vi "svfa_Spectrum Peak Tone Search and Estimation (complex).vi"(8 "error in (no error)":errorcluster, 9 "criterion":T1={"Single/Multiple"=enum."Multiple Peaks", "Threshold"=0.0, "advanced search"={"approximate frequencies"=[], "advanced span [Hz]"=5.0}} {"advanced search"."advanced span [Hz]" format="%0.2p"; "Threshold" format="%.2f"}, 11 "complex spectrum":T9={"complex spectrum response"={"f0"=0.0, "df"=1.0, "complex spectrum"=[]}, "spectrum info"={"channel name"="", "description"="", "x-axis units"=0, "spectral info"={"spectrum type"=enum."Power [Magnitude^2]", "linear/dB"=enum."linear", "window"=0, "window size"=0, "FFT size"=0}, "engineering units"=0, "custom label"="", "dB reference [EU]"=0.0, "peak units"=enum."rms", "weighting filter"=0, "spectral density?"=FALSE, "unit label"="", "spectrum skewed?"=FALSE, "complimentary spectrum units"=enum."none"}} {"spectrum info"."x-axis units" items=["Time (s)"=0, "Frequency-CB (Hz)"=1, "Frequency-CPB (Hz)"=1248, "Frequency-Arbitrary (Hz)"=2357, "Quefrency (s)"=2, "Revolutions (rev)"=3, "Order"=4, "Speed (RPM)"=11, "Speed (rad/s)"=21, "Index"=65535]; "spectrum info"."weighting filter" items=["Linear", "A-weighting", "B-weighting", "C-weighting", "ITU-R 468-4", "Dolby", "CCITT", "C-message", "Wb", "Wc", "Wd", "We", "Wf", "Wh", "Wj", "Wk", "Wm", "AES17 20 kHz lowpass", "AES17 40 kHz lowpass", "AES17 20 kHz highpass", "AES17 40 kHz highpass"]; "spectrum info"."dB reference [EU]" format="%.2f"; "spectrum info"."engineering units" items=["custom..."=0, "V"=1, "A"=21, "C"=30, "pC"=31, "s"=32, "-"=29, "Pa"=2, "N"=20, "g"=3, "m/s^2"=4, "m/s"=5, "m"=6, "mm/s"=12, "mm"=13, "micron/s"=14, "micron"=15, "in/s^2"=7, "in/s"=8, "in"=9, "mil/s"=10, "mil"=11, "rad/s^2"=16, "rad/s"=17, "rad"=18, "deg/s^2"=26, "deg/s"=27, "deg"=28, "RPM"=22, "cycle/s^2"=23, "Hz"=24, "cycle"=25, "strain"=19]; "spectrum info"."spectral info"."window" items=["None "=0, "Hanning"=1, "Hamming"=2, "Blackman-Harris"=3, "Exact Blackman"=4, "Blackman"=5, "Flat Top"=6, "4 Term B-Harris "=7, "7 Term B-Harris"=8, "Low Sidelobe"=9, "Force - Exponential"=10, "Gaussian"=62]; "complex spectrum response"."complex spectrum" format="%.2f"; "complex spectrum response"."df" format="%.9f"; "complex spectrum response"."f0" format="%.2f"}) -> (0 "error out":errorcluster, 2 "Number of peaks":i32, 3 "peaks":T2(array[cluster]) {"phase [degree]" format="%.2f"; "magnitude" format="%.4f"; "frequency [Hz]" format="%.2f"})   [LabVIEW 2017]
uses:
  <vilib>/addons/_NISVFA/_Shared subVIs/Controls/svc_Spectrum Info.ctl
  <vilib>/addons/_NISVFA/_Shared subVIs/Controls/svc_X-Axis Units.ctl
  <vilib>/addons/_NISVFA/_Shared subVIs/Controls/svc_Spectrum Type.ctl
  <vilib>/addons/_NISVFA/_Shared subVIs/Controls/svc_Engineering Units Text Ring.ctl
  <vilib>/addons/_NISVFA/_Shared subVIs/Controls/svc_Weighting Filter Text Ring.ctl
  <vilib>/addons/_NISVFA/_Shared subVIs/Controls/svc_Complimentary Spectrum Units.ctl
  <vilib>/Analysis/_algsub.llb/Vector Norm.vi
  <vilib>/Analysis/_algsub.llb/Complex Vector Norm.vi
  <vilib>/addons/_NISVFA/_Spectrum Processing/subVIs/svfa_Tone Estimation (complex).vi
  <vilib>/addons/_NISVFA/_Spectrum Processing/SVFA Get Spectrum Subset.vi
  <vilib>/addons/_NISVFA/_Spectrum Processing/SVFA Get Spectrum Subset (Complex) (1 Ch).vi
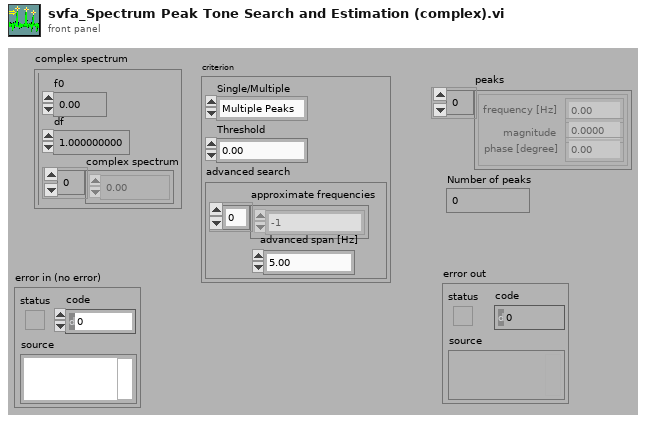
[diagram p1: front panel]
types:
  T1 = cluster{"Single/Multiple":enum16{"Multiple Peaks", "Single Max Peak"}, "Threshold":dbl, "advanced search":cluster{"approximate frequencies":dbl[], "advanced span [Hz]":dbl}}
  T2 = cluster{"frequency [Hz]":dbl, "magnitude":dbl, "phase [degree]":dbl}[]
  T3 = typedef "svc_Spectrum Info.ctl" = cluster{"channel name":string, "description":string, "x-axis units":T4, "spectral info":cluster{"spectrum type":T5, "linear/dB":enum16{"linear", "dB"}, "window":u16, "window size":i32, "FFT size":i32}, "engineering units":T6, "custom label":string, "dB reference [EU]":dbl, "peak units":enum16{"rms", "peak", "peak-peak"}, "weighting filter":T7, "spectral density?":bool, "unit label":string, "spectrum skewed?":bool, "complimentary spectrum units":T8}
  T4 = typedef "svc_X-Axis Units.ctl" = u16
  T5 = typedef "svc_Spectrum Type.ctl" = enum16{"FFT Spectrum [complex]", "Amplitude [Magnitude]", "Power [Magnitude^2]", "Cross Spectrum [complex]", "Frequency Response [Complex]"}
  T6 = typedef "svc_Engineering Units Text Ring.ctl" = u16
  T7 = typedef "svc_Weighting Filter Text Ring.ctl" = u16
  T8 = typedef "svc_Complimentary Spectrum Units.ctl" = enum16{"none", "radians", "degrees", "cycles", "imaginary"}
  T9 = cluster{"complex spectrum response":cluster{"f0":dbl, "df":dbl, "complex spectrum":cdb[]}, "spectrum info":T3}
  T10 = cluster{"frequency [Hz]":dbl, "amplitude":dbl, "phase [degree]":dbl}[]
  T11 = cluster{"frequency [Hz]":dbl, "amplitude":dbl, "phase [degree]":dbl}
  T12 = cluster{"frequency":dbl, "amplitude":dbl, "phase [degree]":dbl}
  T13 = cluster{"frequency [Hz]":dbl, "amplitude [EU pk]":dbl, "phase [deg]":dbl}
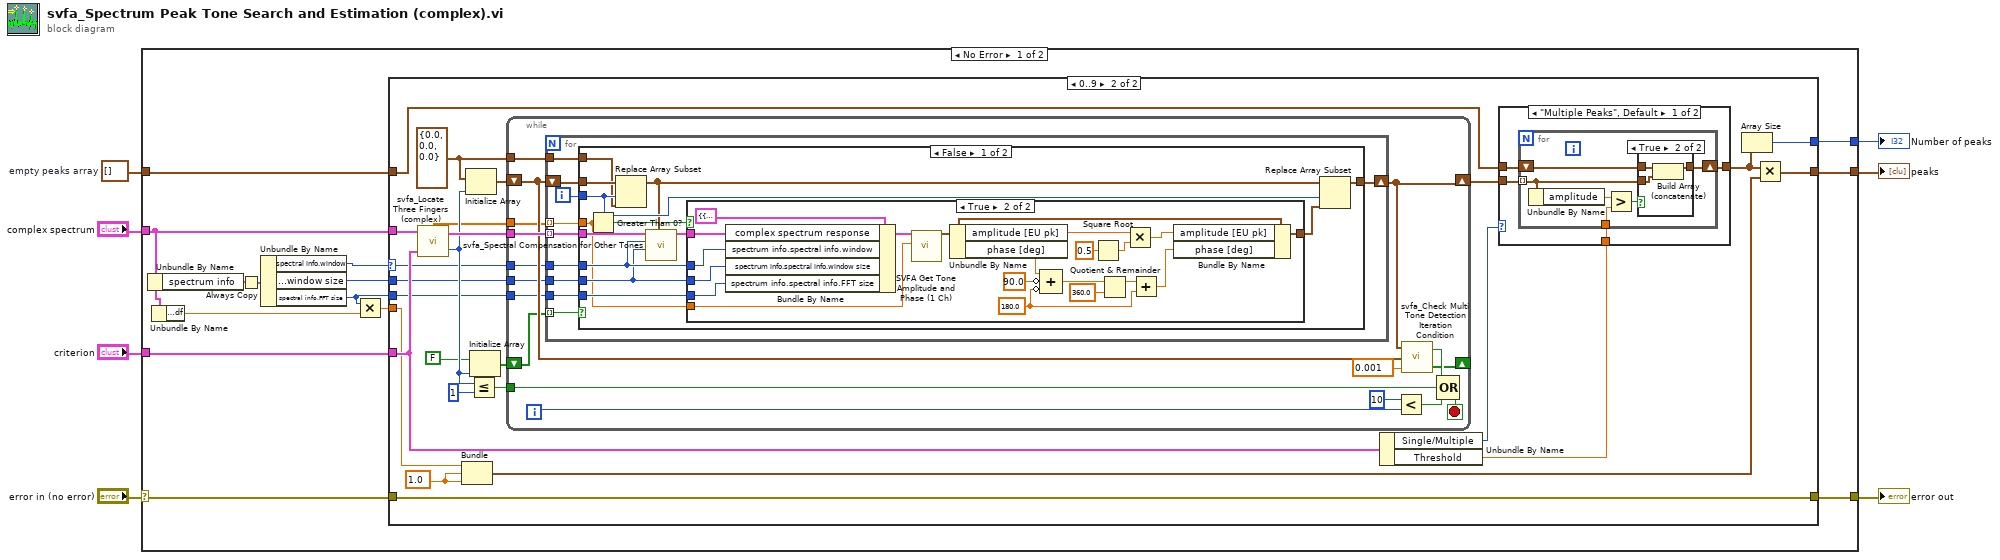
[diagram p0: block diagram]
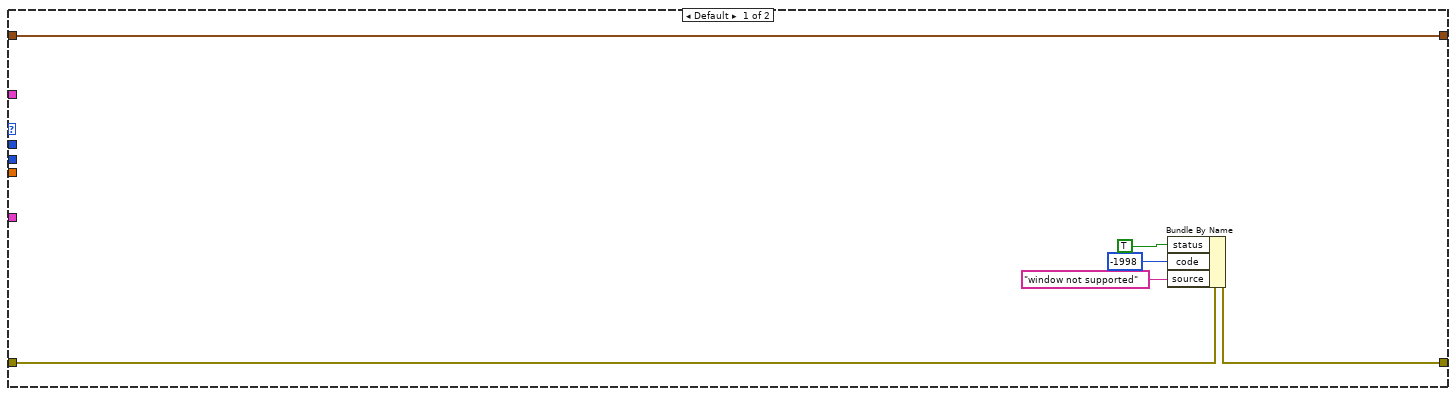
[diagram p2: hidden frame]
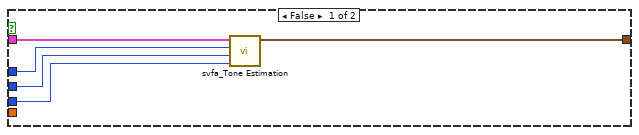
[diagram p3: hidden frame]
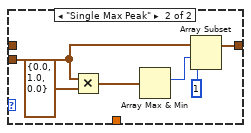
[diagram p6: hidden frame]
diagram:
  w1 = T10 []  # empty peaks array
  n1 = case shown="No Error" "error in (no error)" {
    selector: "error in (no error)" -> [w17 w140]
    tunnel: [w16 w140] -> w6
    tunnel: "criterion" -> [w8 _]
    tunnel: "complex spectrum" -> [w12 _]
    tunnel: [w20 w139] -> w3
    tunnel: [w19 _] -> w2
    tunnel: w1 -> [w9 w139]
    frame No Error {
      n2 = Unbundle By Name(w12) -> ("spectrum info"=w13:T3)
      n3 = Unbundle By Name(w12) -> ("complex spectrum response.df"=w11:dbl)
      n4 = Always Copy(1:w13) -> (0:w10:T3)
      n5 = Unbundle By Name(w10) -> ("spectral info.window"=w18:u16, "spectral info.window size"=w21:i32, "spectral info.FFT size"=w15:i32)
      n6 = Multiply(x=w15, y=w11) -> (x*y=w14:dbl)
      n7 = case shown="0..9" w18 {
        selector: w18 -> [_ w32]
        tunnel: w12 -> [_ w39]
        tunnel: w8 -> [_ w38]
        tunnel: w21 -> [_ w36]
        tunnel: w15 -> [_ w35]
        tunnel: [w22 w34] -> w20
        tunnel: [_ w33] -> w19
        tunnel: w17 -> [w27 w31]
        tunnel: [w23 w31] -> w16
        tunnel: w14 -> [_ w30]
        tunnel: w9 -> [w22 w29]
        frame Default {
          n8 = Bundle By Name(cluster=w27, "status"=TRUE, "code"=-1998, "source"="window not supported") -> (w23:errorcluster)
        }
        frame 0..9 {
          w37 = T11 {"frequency [Hz]"=0.0, "amplitude"=0.0, "phase [degree]"=0.0} ("single tone info.")
          w47 = 1.0 ("x*y")
          n9 = call <vilib>:"svfa_Locate Three Fingers (complex).vi"("criterion"=w38, "complex spectrum"=w39) -> ("number of tones"=w42:i32, "three fingers (frequency normorlized)"=w52:cluster{"f0":dbl, "df":dbl, "spectrum":cdb[]}[], "exact normalized frequencies?"=w28:dbl[])  [unwired: 1 in]
          n10 = Bundle(w30, "x*y"=w47, "x*y"=w47) -> (w48:cluster{dbl, "x*y":dbl, "x*y":dbl})  [unwired: 1 in]
          n11 = Initialize Array(w37, w42) -> (w51:T10)
          n12 = Less Or Equal?(x=w42, y=1) -> (x <= y?=w49:bool)
          n13 = Initialize Array(FALSE ("all stable?"), w42) -> (w43:bool[])
          n14 = while {
            shift-left: w43 -> [w59]
            shift-right: [w58] -> _
            tunnel: w49 -> [w65]
            shift-left: w51 -> [w67]
            shift-right: [w68] -> w46
            tunnel: w52 -> [w69]
            tunnel: w37 -> [w57]
            tunnel: w32 -> [w56]
            tunnel: w36 -> [w55]
            tunnel: w35 -> [w54]
            tunnel: w28 -> [w53]
            i -> [w63]
            stop <- w61 stop-if-true
            n15 = for {
              tunnel: w69 -> [w78] mode=indexing
              shift-right: [w79] -> w68
              shift-left: w67 -> [w77]
              tunnel: w59 -> [w75] mode=indexing
              tunnel: w57 -> [w74]
              tunnel: w56 -> [w73]
              tunnel: w55 -> [w72]
              tunnel: w54 -> [w71]
              tunnel: w53 -> [w70] mode=indexing
              i -> [w76]
              n16 = case shown="False" w75 {
                tunnel: [w92 w118] -> w79
                tunnel: w78 -> [w91 _]
                tunnel: w77 -> [w90 w118]
                tunnel: w76 -> [w89 _]
                tunnel: w74 -> [w86 _]
                tunnel: w73 -> [w84 _]
                tunnel: w72 -> [w83 _]
                tunnel: w71 -> [w82 _]
                tunnel: w70 -> [w80 _]
                frame False {
                  n17 = Greater Than 0?(x=w80) -> (x > 0?=w81:bool)
                  n18 = Replace Array Subset(array=w90, new element=w86, index=w89) -> (w85:T10)
                  n19 = call <vilib>:"svfa_Spectral Compensation for Other Tones.vi"("other tones' information"=w85, "window size"=w83, "window"=w84, "FFT spectrum"=w91) -> ("compensated FFT spectrum"=w88:cluster{"f0":dbl, "df":dbl, "spectrum":cdb[]})  [unwired: 7 in]
                  n20 = case shown="True" w81 {
                    tunnel: w88 -> [w97 w116]
                    tunnel: [w96 w109] -> w87
                    tunnel: w84 -> [w95 w115]
                    tunnel: w83 -> [w94 w114]
                    tunnel: w82 -> [w93 w113]
                    tunnel: w80 -> [_ w111]
                    frame False {
                      n21 = call-poly <vilib>:"svfa_Tone Estimation.vi"("FFT size"=w93, "window size"=w94, "window"=w95, "three fingers"=w97) -> ("single tone info."=w96:T12)  [unwired: 7 in]
                    }
                    frame True {
                      w103 = 180.0 ("x")
                      n22 = Bundle By Name(cluster=T9 {"complex spectrum response"={"f0"=0.0, "df"=1.0, "complex spectrum"=[]}, "spectrum info"={"channel name"="", "description"="", "x-axis units"=0, "spectral info"={"spectrum type"=enum."Power [Magnitude^2]", "linear/dB"=enum."linear", "window"=0, "window size"=0, "FFT size"=0}, "engineering units"=0, "custom label"="", "dB reference [EU]"=0.0, "peak units"=enum."rms", "weighting filter"=0, "spectral density?"=FALSE, "unit label"="", "spectrum skewed?"=FALSE, "complimentary spectrum units"=enum."none"}} ("complex spectrum"), "complex spectrum response"=w116, "spectrum info.spectral info.window"=w115, "spectrum info.spectral info.window size"=w114, "spectrum info.spectral info.FFT size"=w113) -> (w112:T9)
                      n23 = call <vilib>:"SVFA Get Tone Amplitude and Phase (1 Ch).vi"("complex spectrum"=w112, "tone frequency [Hz]"=w111) -> ("identified tone"=w110:T13)  [unwired: 16 in, 1 out]
                      n24 = Unbundle By Name(w110) -> ("amplitude [EU pk]"=w100:dbl, "phase [deg]"=w108:dbl)
                      n25 = Compound Arithmetic op=ADD(w108, invert 90.0 ("x"), invert w103) -> (w106:dbl)
                      n26 = Square Root(x=0.5 ("Input")) -> (sqrt(x)=w99:dbl)
                      n27 = Quotient & Remainder(x=w106, y=360.0 ("x")) -> (x-y*floor(x/y)=w104:dbl)  [unwired: 1 out]
                      n28 = Multiply(x=w100, y=w99) -> (x*y=w98:dbl)
                      n29 = Add(x=w104, y=w103) -> (x+y=w102:dbl)
                      n30 = Bundle By Name(cluster=w110, "amplitude [EU pk]"=w98, "phase [deg]"=w102) -> (w109:T13)
                    }
                  }
                  n31 = Replace Array Subset(array=w85, new element=w87, index=w89) -> (w92:T10)
                }
                frame True {
                }
              }
            }
            n32 = Less?(x=10, y=w63) -> (x < y?=w64:bool)
            n33 = call <vilib>:"svfa_Check Multi Tone Detection Iteration Condition.vi"("precision"=0.001, "peaks before"=w67, "peaks after"=w68) -> ("stable?"=w58:bool[], "all stable?"=w66:bool)
            n34 = Compound Arithmetic op=OR(w66, w65, w64) -> (w61:bool)
          }
          n35 = Unbundle By Name(w38) -> ("Single/Multiple"=w40:enum16{"Multiple Peaks", "Single Max Peak"}, "Threshold"=w45:dbl)
          n36 = case shown="\"Multiple Peaks\", Default" w40 {
            tunnel: w46 -> [w122 w136]
            tunnel: w29 -> [w121 _]
            tunnel: w45 -> [w120 _]
            tunnel: [w119 w133] -> w44
            frame "Multiple Peaks", Default {
              n37 = for {
                tunnel: w122 -> [w125] mode=indexing
                shift-right: [w124] -> w119
                shift-left: w121 -> [w126]
                tunnel: w120 -> [w128]
                n38 = Unbundle By Name(w125) -> ("amplitude"=w123:dbl)
                n39 = Greater?(x=w123, y=w128) -> (0:w127:bool)
                n40 = case shown="True" w127 {
                  tunnel: w126 -> [w129 w132]
                  tunnel: w125 -> [_ w131]
                  tunnel: [w129 w130] -> w124
                  frame False {
                  }
                  frame True {
                    n41 = Build Array (concatenate)(w132, w131) -> (w130:T10)
                  }
                }
              }
            }
            frame "Single Max Peak" {
              n42 = Multiply(x=w136, y=T11 {"frequency [Hz]"=0.0, "amplitude"=1.0, "phase [degree]"=0.0} ("single tone info.")) -> (x*y=w137:T10)
              n43 = Array Max & Min(array=w137) -> (max index (indices)=w135:i32)  [unwired: 3 out]
              n44 = Array Subset(array=w136, index=w135, length=1 ("Array Length")) -> (w133:T10)
            }
          }
          n45 = Array Size(array=w44) -> (size(s)=w33:i32)
          n46 = Multiply(x=w44, y=w48) -> (x*y=w34:cluster{dbl, dbl, dbl}[])
        }
      }
    }
    frame Error {
    }
  }
  "error out" <- w6
  "peaks" <- w3
  "Number of peaks" <- w2
